vi "Read Output.vi"(5 "error in (no error)":errorcluster, 8 "VISA resource name":refnum<visa-resource-name>) -> (0 "error out":errorcluster, 1 "Current":dbl, 2 "Voltage":dbl, 3 "VISA resource name out":refnum<visa-resource-name>, 4 "CV Mode?":bool)   [LabVIEW 2019, in "9103Series.lvlib"]
doc: "Returns the actual voltage level and actual current level for a desired channel."
uses:
  <instrlib>/9103Series/9103Series.lvlib
panel:
  out "ok?":string
  out "Raw Data":string
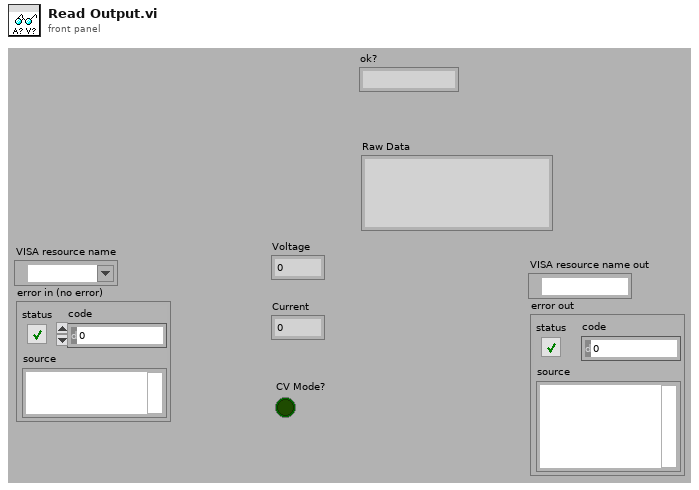
[diagram p1: front panel]
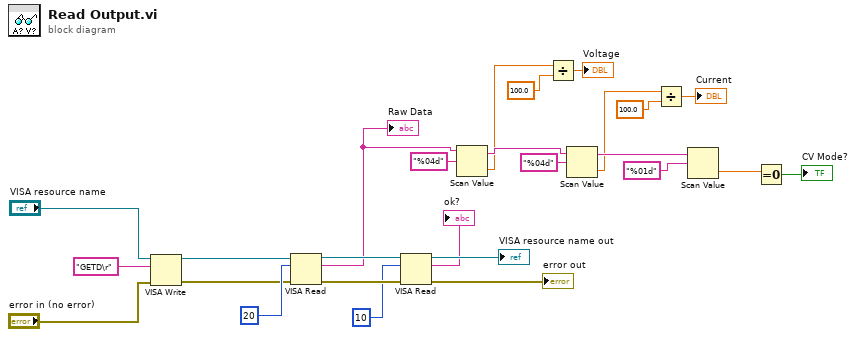
[diagram p0: block diagram]
diagram:
  n1 = VISA Write(VISA resource name="VISA resource name", write buffer="GETD\r", error in (no error)="error in (no error)") -> (VISA resource name out=w22:refnum<visa-resource-name>, error out=w21:errorcluster)  [unwired: 1 out]
  n2 = VISA Read(VISA resource name=w22, byte count=u32 20, error in (no error)=w21) -> (VISA resource name out=w20:refnum<visa-resource-name>, read buffer=w11:string, error out=w19:errorcluster)  [unwired: 1 out]
  "Raw Data" <- w11
  n3 = VISA Read(VISA resource name=w20, byte count=u32 10, error in (no error)=w19) -> (VISA resource name out=→"VISA resource name out":refnum<visa-resource-name>, read buffer=→"ok?":string, error out=→"error out":errorcluster)  [unwired: 1 out]
  n4 = Scan Value(string=w11, format string="%04d") -> (output string=w12:string, value=w2:dbl)  [unwired: 1 in]
  n5 = Divide(x=w2, y=100.0) -> (x/y=→"Voltage":dbl)
  n6 = Scan Value(string=w12, format string="%04d") -> (output string=w10:string, value=w5:dbl)  [unwired: 1 in]
  n7 = Divide(x=w5, y=100.0) -> (x/y=→"Current":dbl)
  n8 = Scan Value(string=w10, format string="%01d") -> (value=w8:dbl)  [unwired: 1 in, 1 out]
  n9 = Equal To 0?(x=w8) -> (x = 0?=→"CV Mode?":bool)
